vi "Proiect RN.vi"() -> ()   [LabVIEW 2024]
panel:
  out "Image":T1(plugin-control)
  in  "File Path":path
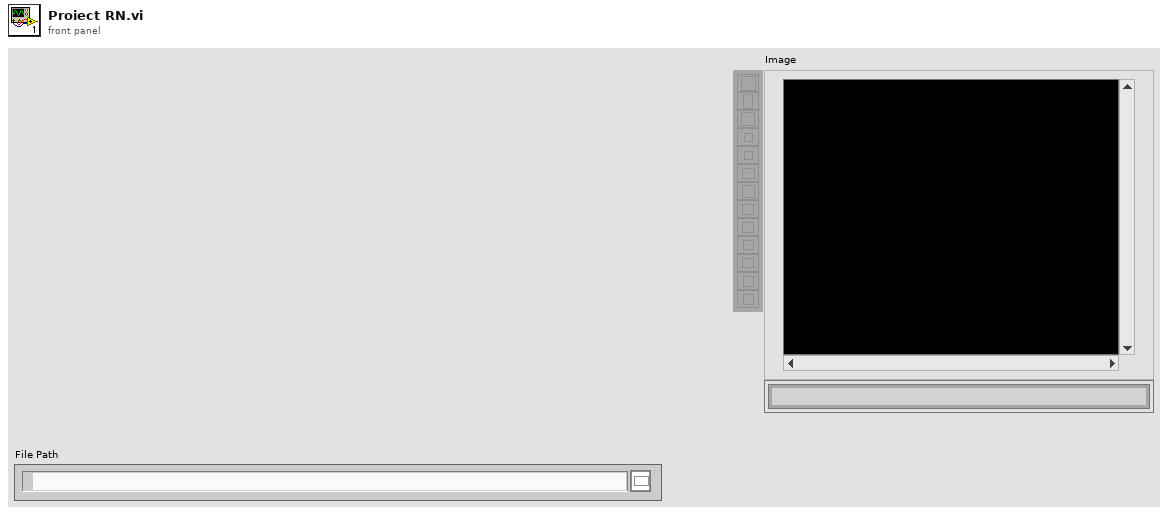
[diagram p1: front panel]
types:
  T1 = typedef "IMAQ Image.ctl" = refnum<image>
  T2 = typedef "Image Type" = u32
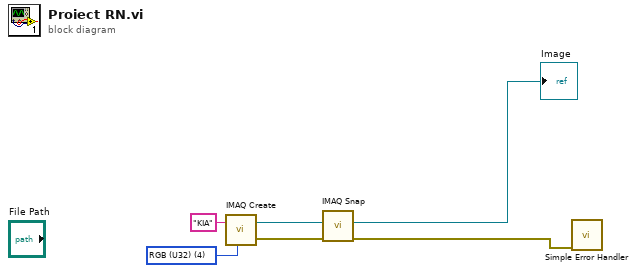
[diagram p0: block diagram]
diagram:
  w4 = T2 4 items=["Grayscale (U8)", "Grayscale (I16)", "Grayscale (SGL)", "Complex (CSG)", "RGB (U32)", "HSL (U32)", "RGB (U64)", "Grayscale (U16)"] ("Image Type")
  n1 = call "IMAQ Create"("Image Name"="KIA", "Image Type"=w4) -> ("New Image"=w5:T1, "error out"=w3:errorcluster)  [unwired: 3 in]
  n2 = call <vilib>:"IMAQ Snap.vi"("error in (no error)"=w3, "Image In"=w5) -> ("error out"=w1:errorcluster, "Image Out"=→"Image":T1)  [unwired: 7 in, 1 out]
  n3 = call <vilib>:"Simple Error Handler.vi"("error in (no error)"=w1) -> ()  [unwired: 4 in, 5 out]
